vi "EndTestSuite_WithFailureAtSiblingSubtree_ParentFailedIconSet.vi"() -> (0 "error out":errorcluster)   [LabVIEW 2019, in "ResultTreeListenerTest.lvlib"]
uses:
  ResultTreeListenerTest.lvlib
  ResultTree/Icon.ctl
  275d98eb-69a7-4435-8809-2af3ffd1cf1d.vi
  Support/FakeTestSuite/FakeTestSuite.lvclass
  C:/Users/de200256/Code/LVUnit/TestSuite/TestSuite.lvclass
  Support/FakeTestCase/FakeTestCase.lvclass
  C:/Users/de200256/Code/LVUnit/TestCase/TestCase/TestCase.lvclass
  Constraint/IsEqual/Create.vi
  ResultTreeListener/ResultTreeListener.lvclass
  Constraint/IsEqual/IsEqual.lvclass
  ResultTree/ResultTree.lvclass
  C:/Users/de200256/Code/LVUnit/Test/Test.lvclass
panel:
  in  "Tree":string(tree)
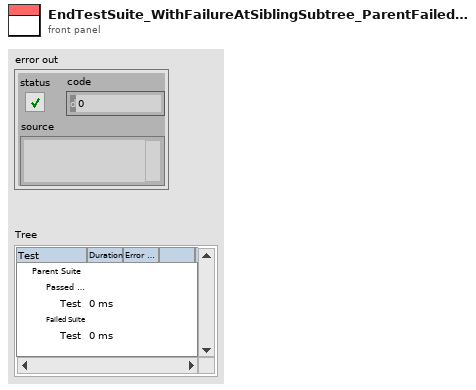
[diagram p1: front panel]
types:
  T1 = typedef "ResultTree.lvclass/Icon.ctl" = enum16{"None", "Passed", "Failed", "Error"}
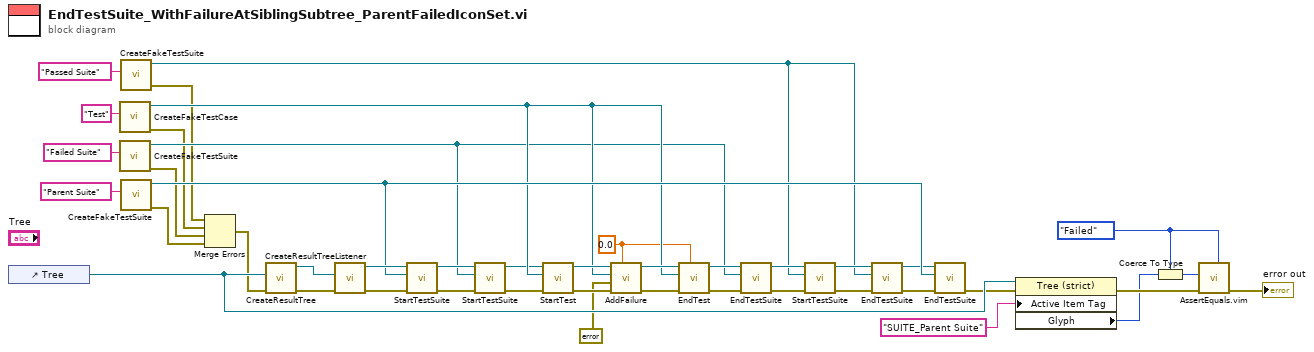
[diagram p0: block diagram]
diagram:
  w20 = 0.0 ("Time")
  w30 = Icon."Failed" ("Active Cell:String")
  n1 = control-ref of="Tree"() -> (w34:refnum<vi>)
  n2 = call "CreateFakeTestCase.vi"("Name"="Test") -> ("error out"=w3:errorcluster, "FakeTestCase out"=w21:refnum<class "FakeTestCase.lvclass">)  [unwired: 9 in]
  n3 = call "CreateFakeTestSuite.vi"("Name"="Failed Suite") -> ("error out"=w2:errorcluster, "FakeTestSuite out"=w11:refnum<class "FakeTestSuite.lvclass">)  [unwired: 9 in]
  n4 = call "CreateFakeTestSuite.vi"("Name"="Passed Suite") -> ("error out"=w4:errorcluster, "FakeTestSuite out"=w8:refnum<class "FakeTestSuite.lvclass">)  [unwired: 9 in]
  n5 = call "CreateFakeTestSuite.vi"("Name"="Parent Suite") -> ("error out"=w1:errorcluster, "FakeTestSuite out"=w36:refnum<class "FakeTestSuite.lvclass">)  [unwired: 9 in]
  n6 = Merge Errors(w4, w3, w2, w1) -> (w29:errorcluster)
  n7 = call "CreateResultTree.vi"("error in (no error)"=w29, "Tree Refnum"=w34) -> ("error out"=w43:errorcluster, "ResultTree out"=w42:refnum<class "ResultTree.lvclass">)  [unwired: 8 in]
  n8 = call "CreateResultTreeListener.vi"("error in (no error)"=w43, "ResultTree"=w42) -> ("error out"=w41:errorcluster, "ResultTreeListener out"=w39:refnum<class "ResultTreeListener.lvclass">)  [unwired: 8 in]
  n9 = call-dynamic "StartTestSuite.vi"("error in (no error)"=w41, "TestSuite"=w36, "ResultTreeListener in"=w39) -> ("error out"=w37:errorcluster, "ResultTreeListener out"=w14:refnum<class "ResultTreeListener.lvclass">)  [unwired: 7 in]
  n10 = call-dynamic "StartTestSuite.vi"("error in (no error)"=w37, "TestSuite"=w11, "ResultTreeListener in"=w14) -> ("error out"=w15:errorcluster, "ResultTreeListener out"=w13:refnum<class "ResultTreeListener.lvclass">)  [unwired: 7 in]
  n11 = call-dynamic "StartTest.vi"("error in (no error)"=w15, "TestCase"=w21, "ResultTreeListener in"=w13) -> ("error out"=w26:errorcluster, "ResultTreeListener out"=w25:refnum<class "ResultTreeListener.lvclass">)  [unwired: 7 in]
  n12 = call-dynamic "AddFailure.vi"("Time"=w20, "error in (no error)"=w26, "Failure"=errorcluster {"status"=TRUE, "code"=1, "source"="Error."}, "TestCase"=w21, "ResultTreeListener in"=w25) -> ("error out"=w27:errorcluster, "ResultTreeListener out"=w22:refnum<class "ResultTreeListener.lvclass">)  [unwired: 5 in]
  n13 = call-dynamic "EndTest.vi"("Time"=w20, "error in (no error)"=w27, "TestCase"=w21, "ResultTreeListener in"=w22) -> ("error out"=w23:errorcluster, "ResultTreeListener out"=w12:refnum<class "ResultTreeListener.lvclass">)  [unwired: 6 in]
  n14 = call-dynamic "EndTestSuite.vi"("error in (no error)"=w23, "TestSuite"=w11, "ResultTreeListener in"=w12) -> ("error out"=w9:errorcluster, "ResultTreeListener out"=w10:refnum<class "ResultTreeListener.lvclass">)  [unwired: 7 in]
  n15 = call-dynamic "StartTestSuite.vi"("error in (no error)"=w9, "TestSuite"=w8, "ResultTreeListener in"=w10) -> ("error out"=w18:errorcluster, "ResultTreeListener out"=w17:refnum<class "ResultTreeListener.lvclass">)  [unwired: 7 in]
  n16 = call-dynamic "EndTestSuite.vi"("error in (no error)"=w18, "TestSuite"=w8, "ResultTreeListener in"=w17) -> ("error out"=w7:errorcluster, "ResultTreeListener out"=w6:refnum<class "ResultTreeListener.lvclass">)  [unwired: 7 in]
  n17 = call-dynamic "EndTestSuite.vi"("error in (no error)"=w7, "TestSuite"=w36, "ResultTreeListener in"=w6) -> ("error out"=w5:errorcluster)  [unwired: 7 in, 1 out]
  n18 = property class="Tree (strict)"(reference=w34, error in=w5, "Active Item Tag"="SUITE_Parent Suite" ("Active Item:Tag")) -> (error out=w35:errorcluster, "Glyph"=w32:i32)  [unwired: 1 out]
  n19 = Coerce To Type(0:w32, 1:w30) -> (2:w31:T1)
  n20 = call "AssertEquals.vim"("Expected"=w30, "error in (no error)"=w35, "Actual"=w31) -> ("error out"=→"error out":errorcluster)  [unwired: 8 in]
